vi "corrigate_measurement_data_by_calibration_coefficients.vi"(8 "Error in":errorcluster, 9 "Offset coeficient":dbl, 10 "Scale coefficient":dbl, 11 "Measurement value":dbl) -> (0 "Error out":errorcluster, 3 "Corrigated measurement value":dbl)   [LabVIEW 2019]
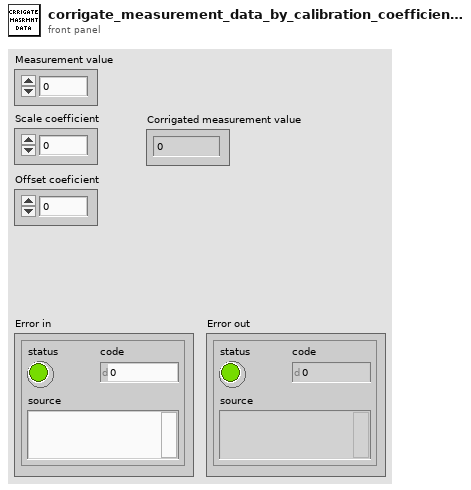
[diagram p1: front panel]
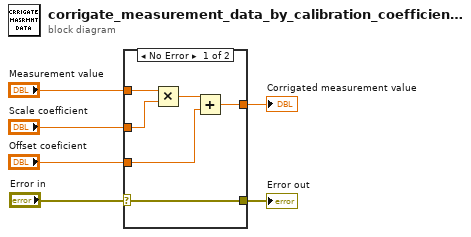
[diagram p0: block diagram]
diagram:
  n1 = case shown="No Error" "Error in" {
    selector: "Error in" -> [w12 w13]
    tunnel: [w12 w13] -> w5
    tunnel: "Measurement value" -> [w11 w14]
    tunnel: "Scale coefficient" -> [w10 _]
    tunnel: "Offset coeficient" -> [w8 _]
    tunnel: [w7 w14] -> w1
    frame No Error {
      n2 = Multiply(x=w11, y=w10) -> (x*y=w9:dbl)
      n3 = Add(x=w9, y=w8) -> (x+y=w7:dbl)
    }
    frame Error {
    }
  }
  "Error out" <- w5
  "Corrigated measurement value" <- w1
